vi "LOC subConvert2DArrayOfStringsToStringList.vi"(1 "InputArray":string[][](array[string])) -> (0 "OutputString":string)   [LabVIEW 2020, in "Localization_Tools.lvlib"]
uses:
  Localization_Tools.lvlib
panel:
  # "VI Name: LOC subConvert2DArrayOfStringsToStringList.vi\nDescription: Converts a 2D array of strings to a list of strings."
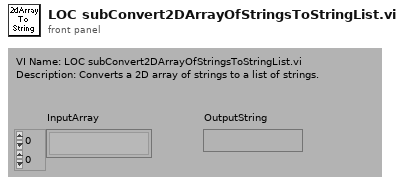
[diagram p1: front panel]
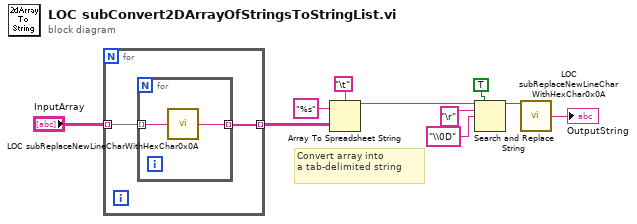
[diagram p0: block diagram]
diagram:
  # "Convert array into\na tab-delimited string"
  n1 = for {
    tunnel: [w12] -> w7 mode=indexing
    tunnel: "InputArray" -> [w11] mode=indexing
    n2 = for {
      tunnel: [w14] -> w12 mode=indexing
      tunnel: w11 -> [w13] mode=indexing
      n3 = call "LOC subReplaceNewLineCharWithHexChar0x0A.vi"("InputString"=w13) -> ("OutputString"=w14:string)
    }
  }
  n4 = Array To Spreadsheet String(delimiter (Tab)="\t", array=w7, 3:"%s" ("format string")) -> (spreadsheet string=w2:string)
  n5 = Search and Replace String(replace all?=TRUE ("replace all? (F)"), input string=w2, search string="\r", replace string="\\0D" ("replace string (\"\")")) -> (result string=w1:string)  [unwired: 4 in, 3 out]
  n6 = call "LOC subReplaceNewLineCharWithHexChar0x0A.vi"("InputString"=w1) -> ("OutputString"=→"OutputString":string)
